vi "Query.vi"(8 "error in":errorcluster, 10 "Query":string, 11 "DB-MySQL in":refnum<class "DB-MySQL.lvclass">=refnum) -> (0 "error out":errorcluster, 1 "Packet Metadata":variant, 2 "Return Data":string[][](array[string]), 3 "DB-MySQL out":refnum<class "DB-MySQL.lvclass">, 4 "Field Names":string[](array[string]))   [LabVIEW 2022 SP3, in "hse-db-mysql.lvlib" / "DB-MySQL.lvclass"]
doc: "____\nHAMPEL SOFTWARE ENGINEERING v1.4.0 (2023-12-19 09:52)"
uses:
  DB-MySQL.lvclass
  DB-MySQL.lvclass/DB-MySQL.ctl
  hse-libraries/Source/hse-misc/hse-misc.lvlib
  <vilib>/Hampel Software Engineering/MySQLNetCom/MySQLNetCom.lvlib
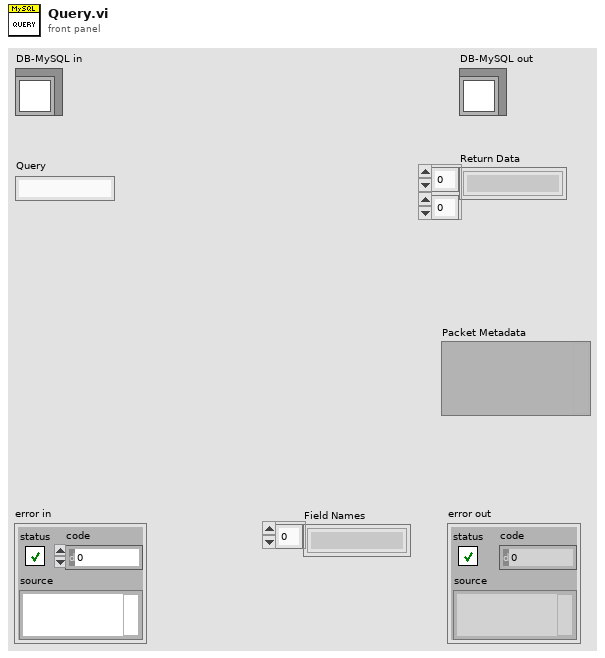
[diagram p1: front panel]
types:
  T1 = typedef "MySQLNetCom.lvlib/OK Packet Metadata.ctl" = cluster{"Affected Rows":u64, "Insert ID":u64, "Server Status":u16, "Warning Count":u16, "Message":string}
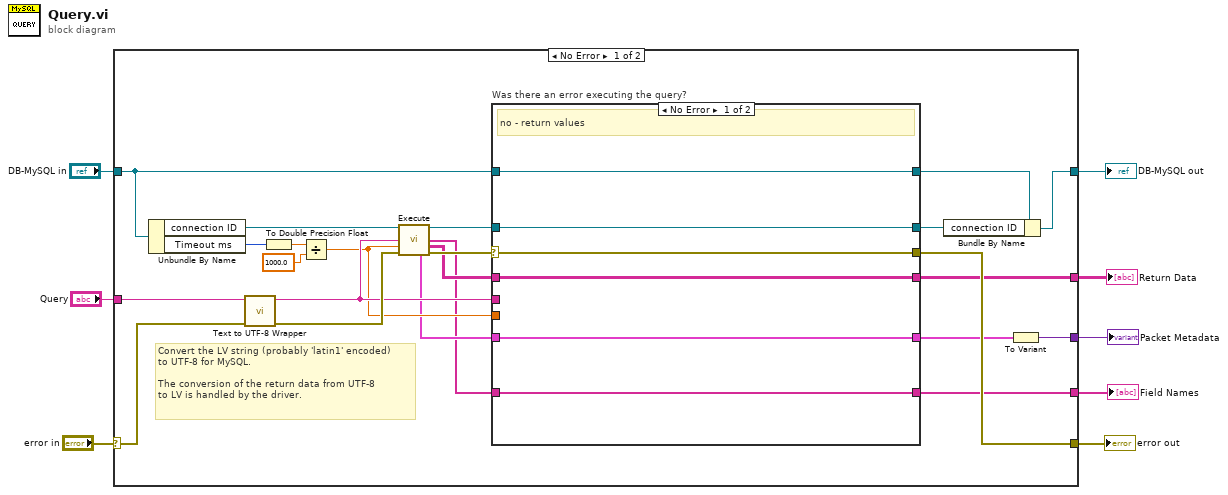
[diagram p0: block diagram]
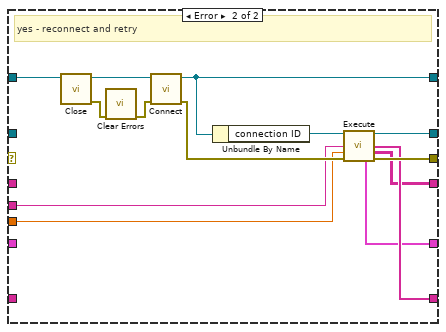
[diagram p2: hidden frame]
diagram:
  n1 = case shown="No Error" "error in" {
    selector: "error in" -> [w17 w52]
    tunnel: "Query" -> [w18 _]
    tunnel: [w30 w53] -> w5
    tunnel: "DB-MySQL in" -> [w25 w53]
    tunnel: [w23 w52] -> w4
    tunnel: [w21 _] -> w2
    tunnel: [w19 _] -> w3
    tunnel: [w26 _] -> w1
    frame No Error {
      # "Convert the LV string (probably 'latin1' encoded)\nto UTF-8 for MySQL.\n\nThe conversion of the return data from UTF-8\nto LV is handled by the driver."
      n2 = Unbundle By Name(w25) -> ("connection ID"=w16:refnum<k5>, "Timeout ms"=w29:i32)
      n3 = call "Text to UTF-8 Wrapper.vi"("error in"=w17, "text"=w18) -> ("error out"=w31:errorcluster, "utf-8 text"=w14:string)  [unwired: 8 in]
      n4 = To Double Precision Float(number=w29) -> (double precision float=w28:dbl)
      n5 = Divide(x=w28, y=1000.0) -> (x/y=w13:dbl)
      n6 = call <vilib>:"Execute.vi"("connection ID in"=w16, "Query"=w14, "Timeout (60s)"=w13, "error in (no error)"=w31) -> ("connection ID out"=w15:refnum<k5>, "Field Names"=w9:string[], "Recordset data out"=w10:string[][], "Packet Metadata"=w12:T1, "error out"=w11:errorcluster)  [unwired: 6 in, 1 out]
      n7 = case "Was there an error executing the query?" shown="No Error" w11 {
        selector: w11 -> [w36 _]
        tunnel: w25 -> [w37 w51]
        tunnel: [w37 w49] -> w24
        tunnel: w10 -> [w34 _]
        tunnel: w12 -> [w33 _]
        tunnel: w9 -> [w32 _]
        tunnel: [w36 w45] -> w23
        tunnel: w15 -> [w35 _]
        tunnel: [w35 w43] -> w22
        tunnel: w14 -> [_ w42]
        tunnel: w13 -> [_ w41]
        tunnel: [w34 w39] -> w21
        tunnel: [w33 w38] -> w20
        tunnel: [w32 w40] -> w19
        frame No Error {
          # "no - return values"
        }
        frame Error {
          # "yes - reconnect and retry"
          n8 = call-dynamic "Close.vi"("DB-MySQL in"=w51) -> ("error out"=w48:errorcluster, "DB-MySQL out"=w50:refnum<class "DB-MySQL.lvclass">)  [unwired: 9 in]
          n9 = call <vilib>:"Clear Errors.vi"("error in (no error)"=w48) -> ("error out"=w47:errorcluster)  [unwired: 5 in, 1 out]
          n10 = call-dynamic "Connect.vi"("error in"=w47, "DB-MySQL in"=w50) -> ("error out"=w46:errorcluster, "DB-MySQL out"=w49:refnum<class "DB-MySQL.lvclass">)  [unwired: 8 in]
          n11 = Unbundle By Name(w49) -> ("connection ID"=w44:refnum<k5>)
          n12 = call <vilib>:"Execute.vi"("connection ID in"=w44, "Query"=w42, "Timeout (60s)"=w41, "error in (no error)"=w46) -> ("connection ID out"=w43:refnum<k5>, "Field Names"=w40:string[], "Recordset data out"=w39:string[][], "Packet Metadata"=w38:T1, "error out"=w45:errorcluster)  [unwired: 6 in, 1 out]
        }
      }
      n13 = Bundle By Name(cluster=w24, "connection ID"=w22) -> (w30:refnum<class "DB-MySQL.lvclass">)
      n14 = To Variant(anything=w20) -> (Variant=w26:variant)
    }
    frame Error {
    }
  }
  "error out" <- w4
  "DB-MySQL out" <- w5
  "Field Names" <- w3
  "Return Data" <- w2
  "Packet Metadata" <- w1
